vi "Folder Tree.vi"(0 "File":path=path "", 1 "Root Folder Name":string="Toolkit") -> (2 "Hierarchy Folders":string[](array[string]))   [LabVIEW 2018, in "Scripts.lvlib"]
uses:
  Scripts.lvlib
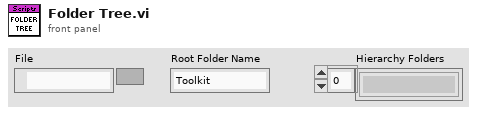
[diagram p1: front panel]
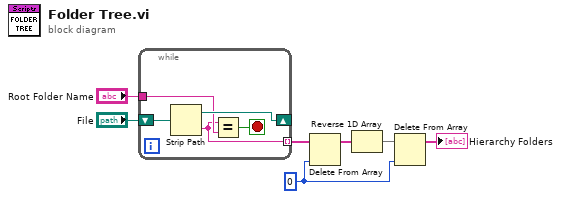
[diagram p0: block diagram]
diagram:
  w1 = 0 ("index")
  n1 = while {
    shift-right: [w11] -> _
    shift-left: "File" -> [w12]
    tunnel: "Root Folder Name" -> [w10]
    tunnel: [w8] -> w5 mode=indexing
    stop <- w9 stop-if-true
    n2 = Strip Path(path=w12) -> (stripped path=w11:path, name=w8:string)
    n3 = Equal?(x=w8, y=w10) -> (x = y?=w9:bool)
  }
  n4 = Delete From Array(array=w5, index=w1) -> (array with subset deleted=w6:string[])  [unwired: 1 in, 1 out]
  n5 = Reverse 1D Array(array=w6) -> (reversed array=w3:string[])
  n6 = Delete From Array(array=w3, index=w1) -> (array with subset deleted=→"Hierarchy Folders":string[])  [unwired: 1 in, 1 out]
